vi "Rename Library.vi"(7 "App":refnum<vi>, 8 "error in (no error)":errorcluster, 10 "New Name":string, 11 "Original Library":path) -> (0 "error out":errorcluster, 1 "Nested Libraries":refnum<vi>[](array[refnum]), 2 "VIs":refnum<vi>[](array[refnum]), 3 "Library":refnum<vi>)   [LabVIEW 2020, in "LV-Protoc.lvlib"]
uses:
  LV-Protoc.lvlib
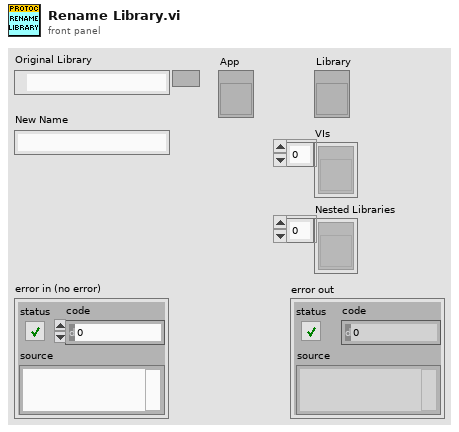
[diagram p1: front panel]
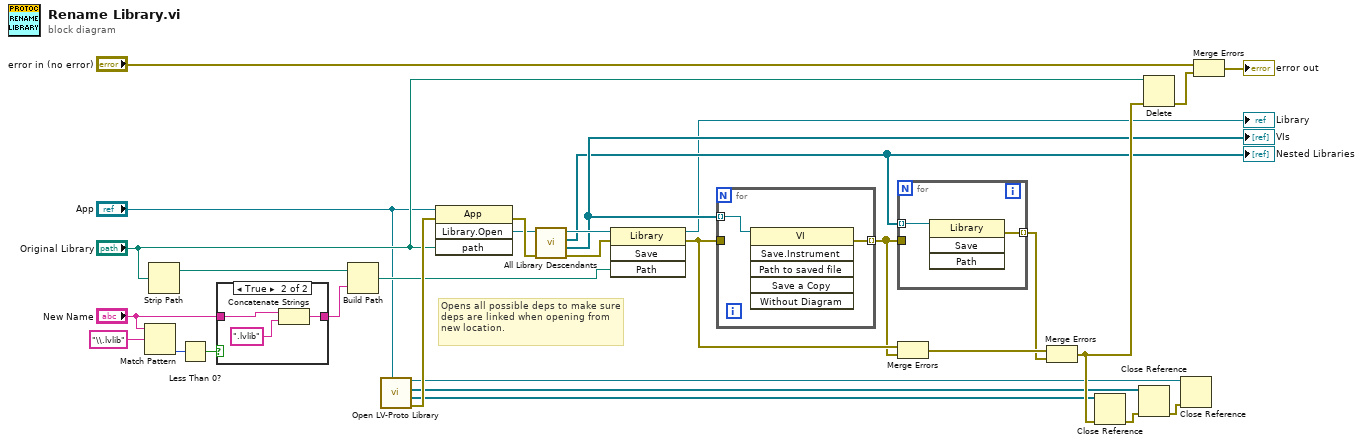
[diagram p0: block diagram]
diagram:
  # "Opens all possible deps to make sure deps are linked when opening from new location."
  n1 = Match Pattern(string="New Name", regular expression="\\.lvlib") -> (offset past match=w26:i32)  [unwired: 1 in, 3 out]
  n2 = Strip Path(path="Original Library") -> (stripped path=w22:path)  [unwired: 1 out]
  n3 = Less Than 0?(x=w26) -> (x < 0?=w25:bool)
  n4 = case shown="True" w25 {
    tunnel: "New Name" -> [w31 w34]
    tunnel: [w31 w32] -> w23
    frame False {
    }
    frame True {
      n5 = Concatenate Strings(w34, ".lvlib" ("string")) -> (w32:string)
    }
  }
  n6 = Build Path(base path=w22, name or relative path=w23) -> (appended path=w28:path)
  n7 = call "Open LV-Proto Library.vi"("App Refnum"="App") -> ("error out"=w29:errorcluster, "VIs"=w10:refnum<vi>[], "Libraries"=w9:refnum<vi>[], "Library"=w6:refnum<vi>)  [unwired: 7 in]
  n8 = invoke class="App" method="Library.Open"(reference="App", error in=w29, "path"="Original Library") -> (error out=w16:errorcluster, "Open Library"=w11:refnum<vi>)  [unwired: 1 in, 2 out]
  n9 = call "All Library Descendants.vi"("error in (no error)"=w16, "Library in"=w11) -> ("error out"=w14:errorcluster, "VIs"=w13:refnum<vi>[], "Libraries"=w12:refnum<vi>[], "Library"=w15:refnum<vi>)  [unwired: 6 in]
  "Nested Libraries" <- w12
  "VIs" <- w13
  n10 = invoke class="Library" method="Save"(reference=w15, error in=w14, "Path"=w28) -> (reference out=→"Library":refnum<vi>, error out=w17:errorcluster)  [unwired: 1 in, 2 out]
  n11 = for {
    tunnel: w13 -> [w36] mode=indexing
    tunnel: w17 -> [_]
    tunnel: [w35] -> w2 mode=indexing
    n12 = invoke class="VI" method="Save.Instrument"(reference=w36) -> (error out=w35:errorcluster)  [unwired: 5 in, 5 out]
  }
  n13 = for {
    tunnel: w12 -> [w38] mode=indexing
    tunnel: [w37] -> w3 mode=indexing
    tunnel: w2 -> [_]
    n14 = invoke class="Library" method="Save"(reference=w38) -> (error out=w37:errorcluster)  [unwired: 3 in, 3 out]
  }
  n15 = Merge Errors(w17, w2) -> (w4:errorcluster)
  n16 = Merge Errors(w4, w3) -> (w30:errorcluster)
  n17 = Close Reference(reference=w10, error in (no error)=w30) -> (error out=w8:errorcluster)
  n18 = Close Reference(reference=w9, error in (no error)=w8) -> (error out=w7:errorcluster)
  n19 = Delete(path (use dialog)="Original Library", error in=w30) -> (error out=w19:errorcluster)  [unwired: 3 in, 2 out]
  n20 = Close Reference(reference=w6, error in (no error)=w7) -> ()  [unwired: 1 out]
  n21 = Merge Errors("error in (no error)", w19) -> (→"error out":errorcluster)
